vi "Mercury_GCS_Sample_Application_2a.vi"(11 "error in":errorcluster) -> (15 "error out":errorcluster)   [LabVIEW 2011]
doc: "This VI demonstrates how to define a Mercury configuration with two Mercury controllers (with GCS firmware) directly connected to the host PC (no DaisyChain) and with stages connected. In this example, the first Mercury is connected through COM port 1 with baudrate 38400 and the second through USB with S/N 1000. The VI runs Mercury_GCS_Configuration_Setup.vi for both controllers with these pre-defined settings and reads the position of the axes. The diagram shows how to combine the driver VIs for these tasks.\nWarning: This VI has Interface settings for each controller that probably do not match your current configuration. Please modify the \"Interface\", \"RS232 settings\" or \"USB settings\" in the diagram before running the VI."
panel:
  in  "stop":bool
  out "Position system 2":dbl[](array[numeric]) format="%.6f"
  out "Identification Mercury controller 2":string
  out "Conn. axes system  2":string[](array[string])
  out "Running":bool caption="Mercury_GCS_Configuration_Setup.vi is running"
  out "Position system 1":dbl[](array[numeric]) format="%.6f"
  out "Conn. axes system 1":string[](array[string])
  out "Identification Mercury controller 1":string
  # "Simple Mercury GCS sample program (two systems, direct connection)"
  # "This VI demonstrates how to define a Mercury configuration with two Mercury controllers (with GCS firmware) directly connected to the host PC (no \nDaisyChain) and with stages connected. In this example, the first Mercury is connected through COM port 1 with baudrate 38400 and the second through \nUSB with S/N 1000. The VI runs Mercury_GCS_Configuration_Setup.vi for both controllers with these pre-defined settings and reads the position of the \naxes. The diagram shows how to combine the driver VIs for these tasks.\n\nWarning: This VI has Interface settings for each controller that probably do not match your current configuration. Please modify the \n                  \"Interface\", \"RS232 settings\" or \"USB settings\" in the diagram before running the VI."
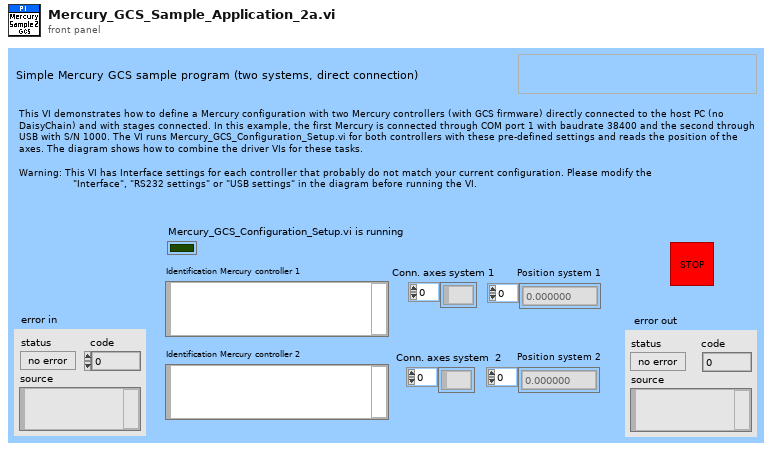
[diagram p1: front panel]
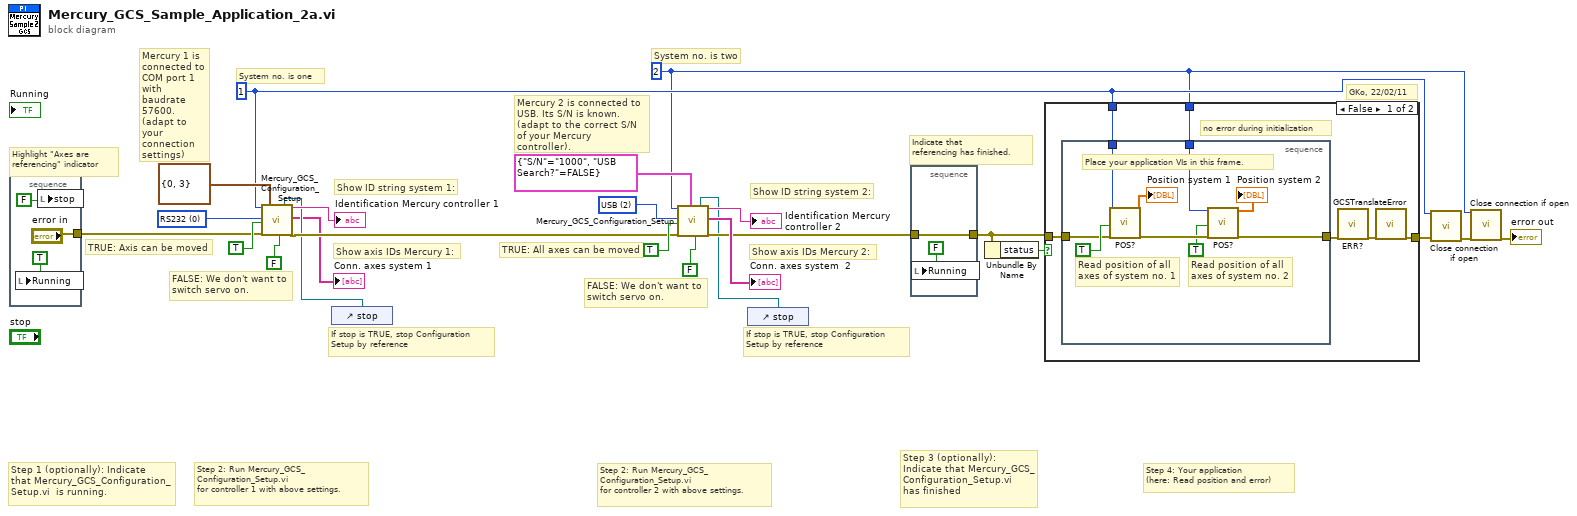
[diagram p0: block diagram]
diagram:
  w1 = u16 2 items=["RS232", "RS232 DaisyChain", "USB", "USB_DaisyChain"] ("Interface")
  w2 = u16 0 items=["RS232", "RS232 DaisyChain", "USB", "USB_DaisyChain"] ("Interface")
  w5 = 2 ("System no.")
  w6 = 1 ("System no.")
  # "Step 4: Your application\n(here: Read position and error)"
  # "Mercury 2 is connected to\nUSB. Its S/N is known.\n(adapt to the correct S/N\nof your Mercury controller)."
  # "Mercury 1 is\nconnected to\nCOM port 1\nwith baudrate\n57600.\n(adapt to your\nconnection\nsettings)"
  # "If stop is TRUE, stop Configuration\nSetup by reference"
  # "If stop is TRUE, stop Configuration\nSetup by reference"
  # "Step 2: Run Mercury_GCS_\nConfiguration_Setup.vi\nfor controller 2 with above settings."
  # "Show axis IDs Mercury 2:"
  # "Show ID string system 2:"
  # "FALSE: We don't want to\nswitch servo on."
  # "TRUE: All axes can be moved"
  # "System no. is two"
  # "GKo, 22/02/11"
  # "Step 3 (optionally): \nIndicate that Mercury_GCS_\nConfiguration_Setup.vi\nhas finished"
  # "Step 2: Run Mercury_GCS_\nConfiguration_Setup.vi\nfor controller 1 with above settings."
  # "Step 1 (optionally): Indicate\nthat Mercury_GCS_Configuration_\nSetup.vi  is running."
  # "Indicate that\nreferencing has finished."
  # "Highlight \"Axes are\nreferencing\" indicator"
  # "Show axis IDs Mercury 1:"
  # "Show ID string system 1:"
  # "FALSE: We don't want to\nswitch servo on."
  # "TRUE: Axis can be moved"
  # "System no. is one"
  n1 = stacked-sequence {
    tunnel: ["error in"] -> w21
    frame #0 {
      n2 = local write "Running"(TRUE ("Running")) -> ()
      n3 = local write "stop"(FALSE ("stop")) -> ()
    }
  }
  n4 = control-ref of="stop"() -> (w14:refnum<vi>)
  n5 = call "Mercury_GCS_Configuration_Setup.vi"("System no."=w6, "Interface"=w2, "All axes?"=TRUE, "error in"=w21, "RS232 settings"=cluster{"Portnumber":i32, "Baudrate":u16} {"Portnumber"=0, "Baudrate"=3}, "Switch servo on?"=FALSE ("Use dialog to define\nconnected stages?"), "Stop refnum"=w14) -> ("Identification"=→"Identification Mercury controller 1":string, "Conn. \nAxes"=→"Conn. axes system 1":string[], "error out"=w16:errorcluster)  [unwired: 6 in, 4 out]
  n6 = control-ref of="stop"() -> (w13:refnum<vi>)
  n7 = call "Mercury_GCS_Configuration_Setup.vi"("System no."=w5, "Interface"=w1, "All axes?"=TRUE, "error in"=w16, "USB settings"=cluster{"S/N":string, "USB Search?":bool} {"S/N"="1000", "USB Search?"=FALSE}, "Switch servo on?"=FALSE ("Use dialog to define\nconnected stages?"), "Stop refnum"=w13) -> ("Identification"=→"Identification Mercury controller 2":string, "Conn. \nAxes"=→"Conn. axes system  2":string[], "error out"=w15:errorcluster)  [unwired: 6 in, 4 out]
  n8 = stacked-sequence {
    tunnel: w15 -> [w29]
    tunnel: [w29] -> w8
    frame #0 {
      n9 = local write "Running"(FALSE ("Running")) -> ()
    }
  }
  n10 = Unbundle By Name(w8) -> ("status"=w9:bool)
  n11 = case shown="False" w9 {
    tunnel: w6 -> [w35 _]
    tunnel: w8 -> [w34 w45]
    tunnel: [w31 w45] -> w7
    tunnel: w5 -> [w30 _]
    frame False {
      # "no error during initialization"
      n12 = stacked-sequence {
        tunnel: w35 -> [w44]
        tunnel: [w38] -> w32
        tunnel: w34 -> [w42]
        tunnel: w30 -> [w36]
        frame #0 {
          # "Read position of all\naxes of system no. 2"
          # "Read position of all \naxes of system no. 1"
          # "Place your application VIs in this frame."
          n13 = call "POS?.vi"("System no."=w44, "All axes?"=TRUE, "error in"=w42) -> ("Position"=→"Position system 1":dbl[], "error out"=w39:errorcluster)  [unwired: 15 in]
          n14 = call "POS?.vi"("System no."=w36, "All axes?"=TRUE, "error in"=w39) -> ("Position"=→"Position system 2":dbl[], "error out"=w38:errorcluster)  [unwired: 15 in]
        }
      }
      n15 = call "ERR?.vi"("error in"=w32) -> ("error out"=w33:errorcluster)  [unwired: 17 in, 1 out]
      n16 = call "GCSTranslateError.vi"("error in"=w33) -> ("error out"=w31:errorcluster)  [unwired: 16 in, 2 out]
    }
    frame True {
      # "error during initialization!"
    }
  }
  n17 = call "Close connection if open.vi"("System no."=w6, "error in"=w7) -> ("error out"=w4:errorcluster)  [unwired: 16 in, 1 out]
  n18 = call "Close connection if open.vi"("System no."=w5, "error in"=w4) -> ("error out"=→"error out":errorcluster)  [unwired: 16 in, 1 out]
